vi "Euler 002.vi"() -> ()   [LabVIEW 2021]
uses:
  <vilib>/Analysis/Matrix/NI_Matrix.lvlib
  <vilib>/Analysis/NI_AALBase.lvlib
  <vilib>/Analysis/7linalg.llb/Real Matrix Power.vi
  <vilib>/Analysis/Matrix/Numeric/Conversions/Array To Matrix - RA2.vi
panel:
  out "Waveform Graph":i32[](graph)
  out "Matrix Eponentiation":i32
  out "Optimized Thirds":i32
  out "Brute Force":i32
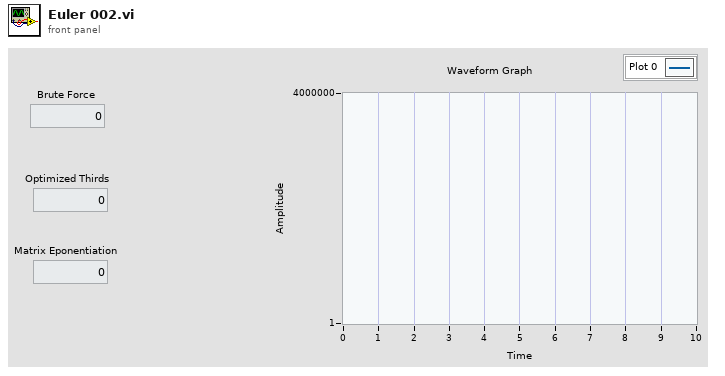
[diagram p1: front panel]
types:
  T1 = typedef "NI_Matrix.lvlib/RealMatrix.ctl" = dbl[][]
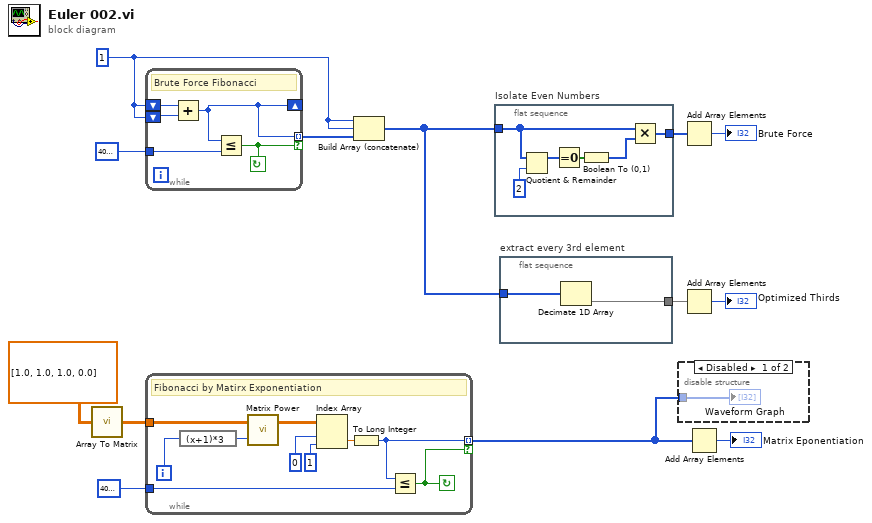
[diagram p0: block diagram]
diagram:
  w3 = 1
  n1 = call-poly <vilib>:"Array To Matrix.vi"("Real 2D Array"=dbl[][] [[1.0, 1.0], [1.0, 0.0]]) -> ("Real Matrix"=w11:T1)
  n2 = while "Brute Force Fibonacci" {
    shift-right: [w15] -> _
    shift-left: w3 -> [w18]
    shift-left: w3 -> [w17]
    tunnel: [w15] -> w6 mode=indexing if=w14
    tunnel: 4000000 ("y") -> [w16]
    stop <- w14 continue-if-true
    # "Brute Force Fibonacci"
    n3 = Add(x=w18, y=w17) -> (x+y=w15:i32)
    n4 = Less Or Equal?(x=w15, y=w16) -> (x <= y?=w14:bool)
  }
  n5 = while "Fibonacci by Matirx Exponentiation" {
    tunnel: w11 -> [w28]
    tunnel: [w21] -> w1 mode=indexing if=w22
    tunnel: 4000000 ("y") -> [w23]
    i -> [w20]
    stop <- w22 continue-if-true
    # "Fibonacci by Matirx Exponentiation"
    n6 = expression code="(x+1)*3"(w20) -> (w19:i32)
    n7 = call-poly <vilib>:"Matrix Power.vi"("n"=w19, "Input Matrix"=w28) -> ("Matrix Power"=w27:T1)  [unwired: 1 out]
    n8 = Index Array(array=w27, index (row)=0 ("index (col)"), index (col)=1) -> (element=w24:dbl)
    n9 = To Long Integer(number=w24) -> (32bit integer=w21:i32)
    n10 = Less Or Equal?(x=w21, y=w23) -> (x <= y?=w22:bool)
  }
  n11 = Build Array (concatenate)(w3, w3, w6) -> (w4:i32[])
  n12 = flat-sequence "Isolate Even Numbers" {
    tunnel: w4 -> [w34]
    tunnel: [w30] -> w5
    frame #0 {
      n13 = Quotient & Remainder(x=w34, y=2) -> (x-y*floor(x/y)=w32:i32[])  [unwired: 1 out]
      n14 = Equal To 0?(x=w32) -> (x = 0?=w31:bool[])
      n15 = Boolean To (0,1)(Boolean=w31) -> (0, 1=w29:i16[])
      n16 = Multiply(x=w34, y=w29) -> (x*y=w30:i32[])
    }
  }
  n17 = flat-sequence "extract every 3rd element" {
    tunnel: w4 -> [w36]
    tunnel: [w35] -> w7
    frame #0 {
      n18 = Decimate 1D Array(w36) -> (w35:i32[])  [unwired: 2 out]
    }
  }
  n19 = disable-structure shown="Disabled" {
    disable-tunnel: w1 -> [w37 _]
    frame Disabled {
      "Waveform Graph" <- w37
    }
    frame Enabled {
    }
  }
  n20 = Add Array Elements(numeric array=w5) -> (sum=→"Brute Force":i32)
  n21 = Add Array Elements(numeric array=w7) -> (sum=→"Optimized Thirds":i32)
  n22 = Add Array Elements(numeric array=w1) -> (sum=→"Matrix Eponentiation":i32)
